vi "DMA Write-FPGA.vi"() -> ()   [LabVIEW 2012]
panel:
  out "Overflow?":bool
  in  "DMA Cleared?":bool
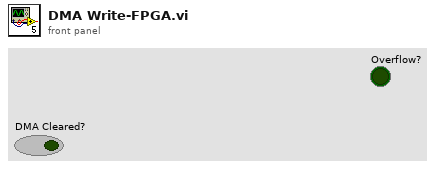
[diagram p1: front panel]
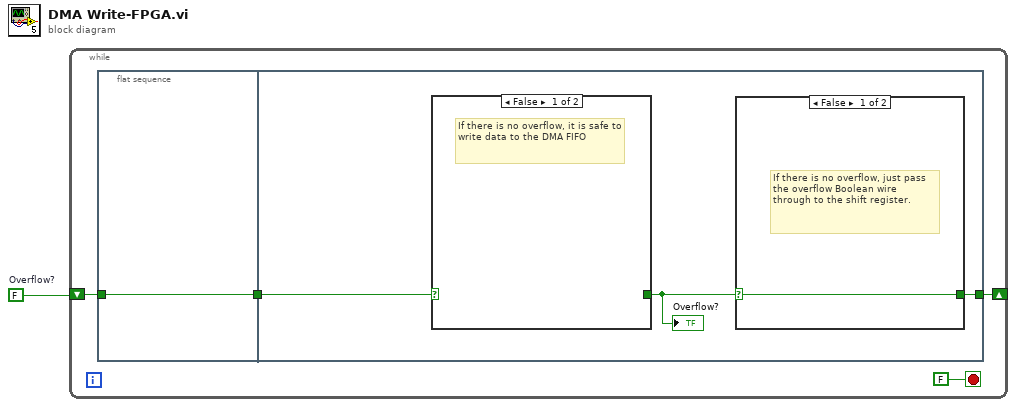
[diagram p0: block diagram]
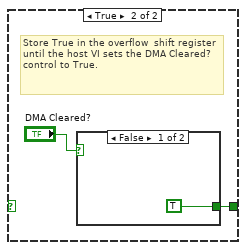
[diagram p3: hidden frame]
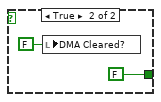
[diagram p4: hidden frame]
diagram:
  w1 = FALSE  # Overflow?
  n1 = while {
    shift-right: [w3] -> _
    shift-left: w1 -> [w4]
    stop <- FALSE stop-if-true
    n2 = flat-sequence {
      tunnel: w4 -> [w6]
      tunnel: [w6] -> w2
      tunnel: [w7] -> w3
      tunnel: w2 -> [w9]
      frame #0 {
      }
      frame #1 {
        n3 = case shown="False" w9 {
          selector: w9 -> [_ w10]
          tunnel: [_ w10] -> w8
          frame False {
            # "If there is no overflow, it is safe to write data to the DMA FIFO"
          }
          frame True {
            # "If there is an overflow, do not write to the DMA FIFO."
          }
        }
        "Overflow?" <- w8
        n4 = case shown="False" w8 {
          selector: w8 -> [w11 _]
          tunnel: [w11 w12] -> w7
          frame False {
            # "If there is no overflow, just pass the overflow Boolean wire through to the shift register."
          }
          frame True {
            # "Store True in the overflow  shift register until the host VI sets the DMA Cleared? control to True."
            n5 = case shown="False" "DMA Cleared?" {
              tunnel: [TRUE FALSE] -> w12
              frame False {
              }
              frame True {
                n6 = local write "DMA Cleared?"(FALSE ("Reset")) -> ()
              }
            }
          }
        }
      }
    }
  }
